vi "MainT4.vi"() -> ()   [LabVIEW 2019]
uses:
  <instrlib>/niDMM/nidmm.llb/niDMM Function.ctl
  <instrlib>/niDMM/nidmm.llb/niDMM Resolution in Digits.ctl
  <extravilib>/ChannelInstances/Tag-bool/Write With Abort.vi
  <extravilib>/ChannelInstances/Tag-bool/Read With Abort.vi
  <extravilib>/ChannelInstances/Tag-bool/Instantiate.vi
  <extravilib>/ChannelInstances/Tag-bool/EndpointRead.vi
  <extravilib>/ChannelInstances/Tag-bool/Endpoint.vi
  <extravilib>/ChannelInstances/Tag-bool.lvlib
panel:
  in  "stop program":bool
  in  "Tab Control":T1(tab)
  out "Waveform Chart 2":cluster{dbl, dbl, dbl}(graph)={9900000000.0, 100000.0, 100000.0}
  in  "Recieve Data":bool=TRUE
  in  "termination char\n(0xA = '\\n' = LF)":u8=13 format="%.0x"
  in  "VISA resource name":refnum<visa-resource-name>="COM3"
  out "time between obtaining data (ms)  (P)":u32
  out "output cluster":cluster{dbl, dbl, dbl}
  out "Waveform Chart 4":T2(graph)
  in  "physical channels":tag="PXI1Slot2/ai0:5"
  in  "resistance configuration":i32(ring)=4 items=["2-Wire"=2, "3-Wire"=3, "4-Wire"=4]
  out "time between obtaining data (ms) (T)":u32
  out "data":dbl[](array[numeric]) format="%0.2f"
  out "Waveform Chart 3":dbl(graph)
  in  "Instrument Descriptor":refnum<k15>="PXI1Slot4"
  in  "Function":T3
  in  "Resolution in Digits":T4=5.5 items=["3 1/2"=3.5, "4 1/2"=4.5, "5 1/2"=5.5, "6 1/2"=6.5, "7 1/2"=7.5]
  in  "Range (Volts)":dbl=10.0 format="%.2p"
  out "Over Range?":bool
  out "time between obtaining data (ms) (v/c)":u32
  out "Measurement (Volts)":dbl caption="Value" format="%_5p"
  in  "Self-Calibrate Multimeter at the beginning?":bool
  # "NEGRO bateria"
  # "BLANCO platina"
  # "VERDE fuente"
  # "AZUL MCU"
  # "AMARILLO AMBIENTE"
  # "ROJO BATERIA RELOJ"
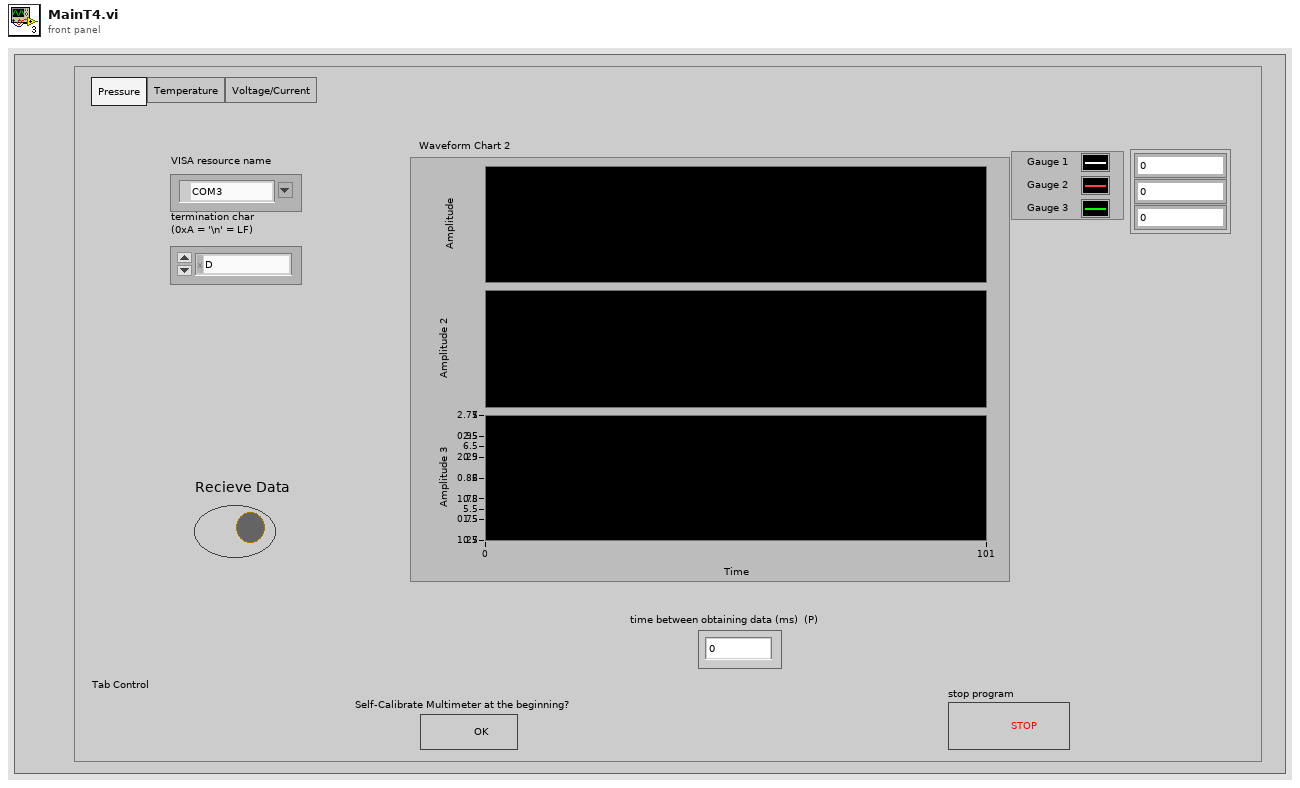
[diagram p1: front panel]
types:
  T1 = enum32{"Pressure", "Temperature", "Voltage/Current"}
  T2 = cluster{"data[0]":dbl, "data[1]":dbl, "data[2]":dbl, "data[3]":dbl, "data[4]":dbl, "data[5]":dbl, "data[6]":dbl, "data[7]":dbl, "data[8]":dbl}
  T3 = typedef "niDMM Function.ctl" = enum16{"DC Volts", "AC Volts", "DC Current", "AC Current", "2-wire Resistance", "4-wire Resistance", "Diode", "Frequency", "Period", "AC Volts DC Coupled", "Capacitance", "Inductance", "Temperature"}
  T4 = typedef "niDMM Resolution in Digits.ctl" = dbl
  T5 = typedef "Tag-bool.lvlib/))Channel.ctl" = refnum<queue>
  T6 = enum16{"open", "replace", "create", "open or create", "replace or create", "replace or create with confirmation"}
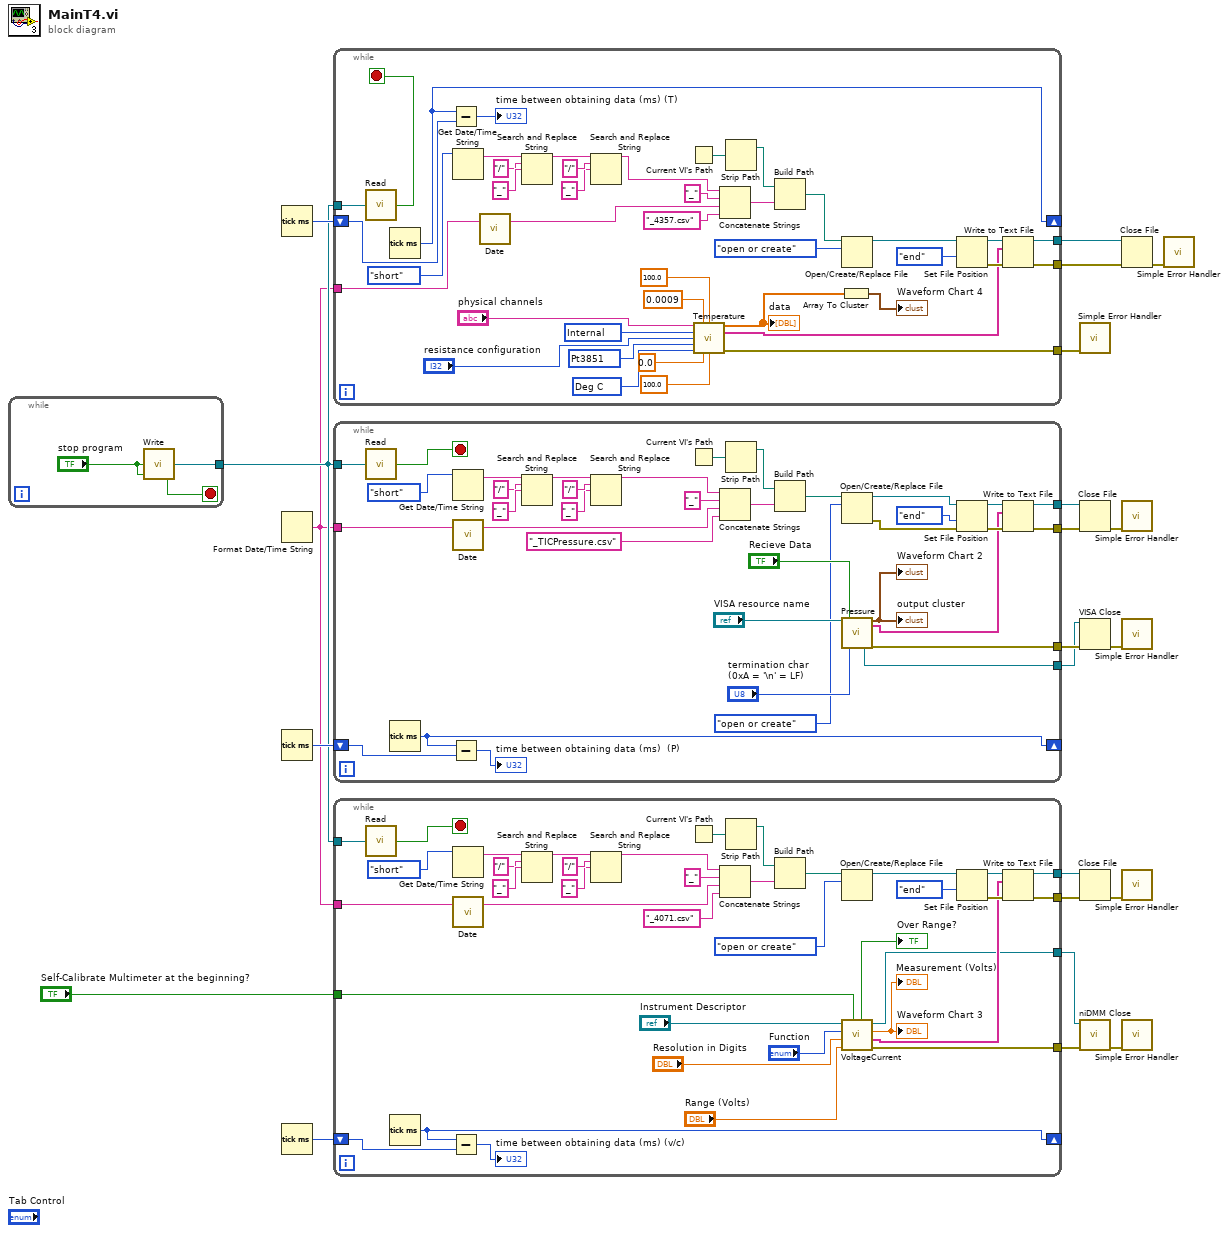
[diagram p0: block diagram]
diagram:
  n1 = while {
    tunnel: [w23] -> w3
    stop <- "stop program" stop-if-true
    n2 = call <extravilib>:"Write.vi"("element"="stop program") -> ("channel"=w23:T5)  [unwired: 1 out]
  }
  n3 = Tick Count (ms)() -> (millisecond timer value=w20:u32)
  n4 = Format Date/Time String() -> (date/time string=w1:string)  [unwired: 3 in]
  n5 = Tick Count (ms)() -> (millisecond timer value=w21:u32)
  n6 = Tick Count (ms)() -> (millisecond timer value=w22:u32)
  n7 = while {
    tunnel: [w48] -> w16
    tunnel: [w47] -> w4
    tunnel: [w46] -> w5
    shift-right: [w43] -> _
    shift-left: w20 -> [w44]
    tunnel: w3 -> [w40]
    tunnel: w1 -> [w28]
    stop <- w39 stop-if-true
    w51 = 10143 items=["Deg C"=10143, "Deg F"=10144, "Kelvins"=10325, "Deg R"=10145, "From Custom Scale"=10065] ("units")
    w52 = 10071 items=["Pt3750"=12481, "Pt3851"=10071, "Pt3911"=12482, "Pt3916"=10069, "Pt3920"=10053, "Pt3928"=12483, "Custom"=10137] ("rtd type")
    w53 = 10200 items=["Internal"=10200, "External"=10167, "None"=10230] ("current excitation source")
    n8 = call <extravilib>:"Read.vi"("channel"=w40) -> ("element"=w39:bool)  [unwired: 1 in, 1 out]
    n9 = Tick Count (ms)() -> (millisecond timer value=w43:u32)
    n10 = Subtract(x=w43, y=w44) -> (x-y=→"time between obtaining data (ms) (T)":u32)
    n11 = Get Date/Time String(date format (0)=enum16{"short", "long", "abbreviated"}."short") -> (date string=w34:string)  [unwired: 2 in, 1 out]
    n12 = call "Date.vi"("Format Date/Time String"=w28) -> ("result string"=w25:string)  [unwired: 2 in]
    n13 = Search and Replace String(input string=w34, search string="/", replace string="_" ("replace string (\"\")")) -> (result string=w37:string)  [unwired: 5 in, 3 out]
    n14 = Search and Replace String(input string=w37, search string="/", replace string="_" ("replace string (\"\")")) -> (result string=w31:string)  [unwired: 5 in, 3 out]
    n15 = Current VI's Path() -> (path=w59:path)
    n16 = call "Temperature.vi"("physical channels"="physical channels", "current excitation value"=0.0009, "r0"=100.0, "current excitation source"=w53, "resistance configuration"="resistance configuration", "rtd type"=w52, "units"=w51, "minimum value"=0.0, "maximum value"=100.0) -> ("data"=w42:dbl[], "output array"=w29:string[], "error out"=w48:errorcluster)  [unwired: 4 in]
    "data" <- w42
    n17 = Concatenate Strings(w31, "_" ("string"), w25, "_4357.csv" ("string")) -> (w30:string)
    n18 = Strip Path(path=w59) -> (stripped path=w58:path)  [unwired: 1 out]
    n19 = Build Path(base path=w58, name or relative path=w30) -> (appended path=w65:path)
    n20 = Array To Cluster(array=w42) -> (cluster=→"Waveform Chart 4":T2)
    n21 = Open/Create/Replace File(file path (use dialog)=w65, operation (0:open)=T6."open or create") -> (refnum out=w62:refnum<file>)  [unwired: 4 in, 2 out]
    n22 = Set File Position(refnum=w62, from (0:start)=enum16{"start", "end", "current"}."end") -> (refnum out=w63:refnum<file>, error out=w64:errorcluster)  [unwired: 2 in]
    n23 = Write to Text File(file (use dialog)=w63, text=w29, error in=w64) -> (refnum out=w47:refnum<file>, error out=w46:errorcluster)  [unwired: 1 in, 1 out]
  }
  n24 = while {
    tunnel: [w87] -> w7
    tunnel: [w86] -> w8
    tunnel: [w85] -> w9
    tunnel: [w84] -> w10
    shift-right: [w81] -> _
    shift-left: w21 -> [w82]
    tunnel: w3 -> [w80]
    tunnel: w1 -> [w69]
    stop <- w79 stop-if-true
    n25 = call <extravilib>:"Read.vi"("channel"=w80) -> ("element"=w79:bool)  [unwired: 1 in, 1 out]
    n26 = Tick Count (ms)() -> (millisecond timer value=w81:u32)
    n27 = Subtract(x=w81, y=w82) -> (x-y=→"time between obtaining data (ms)  (P)":u32)
    n28 = Get Date/Time String(date format (0)=enum16{"short", "long", "abbreviated"}."short") -> (date string=w74:string)  [unwired: 2 in, 1 out]
    n29 = call "Date.vi"("Format Date/Time String"=w69) -> ("result string"=w67:string)  [unwired: 2 in]
    n30 = Search and Replace String(input string=w74, search string="/", replace string="_" ("replace string (\"\")")) -> (result string=w77:string)  [unwired: 5 in, 3 out]
    n31 = Search and Replace String(input string=w77, search string="/", replace string="_" ("replace string (\"\")")) -> (result string=w71:string)  [unwired: 5 in, 3 out]
    n32 = Current VI's Path() -> (path=w90:path)
    n33 = Concatenate Strings(w71, "_" ("string"), w67, "_TICPressure.csv" ("string")) -> (w70:string)
    n34 = Strip Path(path=w90) -> (stripped path=w89:path)  [unwired: 1 out]
    n35 = Build Path(base path=w89, name or relative path=w70) -> (appended path=w97:path)
    n36 = Open/Create/Replace File(file path (use dialog)=w97, operation (0:open)=T6."open or create") -> (refnum out=w94:refnum<file>, error out=w91:errorcluster)  [unwired: 4 in, 1 out]
    n37 = call "Pressure.vi"("VISA resource name"="VISA resource name", "Recieve Data"="Recieve Data", "termination char\n(0xA = '\\n' = LF)"="termination char\n(0xA = '\\n' = LF)") -> ("VISA resource name out"=w87:refnum<visa-resource-name>, "output cluster"=→"Waveform Chart 2" →"output cluster":cluster{dbl, dbl, dbl}, "output array"=w88:string[], "error out"=w86:errorcluster)  [unwired: 10 in, 3 out]
    n38 = Set File Position(refnum=w94, from (0:start)=enum16{"start", "end", "current"}."end", error in=w91) -> (refnum out=w95:refnum<file>, error out=w96:errorcluster)  [unwired: 1 in]
    n39 = Write to Text File(file (use dialog)=w95, text=w88, error in=w96) -> (refnum out=w85:refnum<file>, error out=w84:errorcluster)  [unwired: 1 in, 1 out]
  }
  n40 = while {
    tunnel: "Self-Calibrate Multimeter at the beginning?" -> [w135]
    tunnel: [w123] -> w11
    tunnel: [w122] -> w12
    tunnel: [w121] -> w14
    tunnel: [w120] -> w15
    shift-right: [w117] -> _
    shift-left: w22 -> [w118]
    tunnel: w3 -> [w116]
    tunnel: w1 -> [w105]
    stop <- w115 stop-if-true
    n41 = call <extravilib>:"Read.vi"("channel"=w116) -> ("element"=w115:bool)  [unwired: 1 in, 1 out]
    n42 = Tick Count (ms)() -> (millisecond timer value=w117:u32)
    n43 = Subtract(x=w117, y=w118) -> (x-y=→"time between obtaining data (ms) (v/c)":u32)
    n44 = Get Date/Time String(date format (0)=enum16{"short", "long", "abbreviated"}."short") -> (date string=w110:string)  [unwired: 2 in, 1 out]
    n45 = call "Date.vi"("Format Date/Time String"=w105) -> ("result string"=w103:string)  [unwired: 2 in]
    n46 = Search and Replace String(input string=w110, search string="/", replace string="_" ("replace string (\"\")")) -> (result string=w113:string)  [unwired: 5 in, 3 out]
    n47 = Search and Replace String(input string=w113, search string="/", replace string="_" ("replace string (\"\")")) -> (result string=w107:string)  [unwired: 5 in, 3 out]
    n48 = Current VI's Path() -> (path=w126:path)
    n49 = Concatenate Strings(w107, "_" ("string"), w103, "_4071.csv" ("string")) -> (w106:string)
    n50 = Strip Path(path=w126) -> (stripped path=w125:path)  [unwired: 1 out]
    n51 = Build Path(base path=w125, name or relative path=w106) -> (appended path=w132:path)
    n52 = Open/Create/Replace File(file path (use dialog)=w132, operation (0:open)=T6."open or create") -> (refnum out=w129:refnum<file>)  [unwired: 4 in, 2 out]
    n53 = call "VoltageCurrent.vi"("Self-Calibrate at the beginning?"=w135, "Range (Volts)"="Range (Volts)", "Resolution in Digits"="Resolution in Digits", "Function"="Function", "Instrument Descriptor"="Instrument Descriptor") -> ("error out"=w120:errorcluster, "output array"=w124:string[], "Measurement (Volts)"=→"Waveform Chart 3" →"Measurement (Volts)":dbl, "instrument handle out"=w121:refnum<k15>, "Over Range?"=→"Over Range?":bool)  [unwired: 2 in]
    n54 = Set File Position(refnum=w129, from (0:start)=enum16{"start", "end", "current"}."end") -> (refnum out=w130:refnum<file>, error out=w131:errorcluster)  [unwired: 2 in]
    n55 = Write to Text File(file (use dialog)=w130, text=w124, error in=w131) -> (refnum out=w123:refnum<file>, error out=w122:errorcluster)  [unwired: 1 in, 1 out]
  }
  n56 = call <vilib>:"Simple Error Handler.vi"("error in (no error)"=w16) -> ()  [unwired: 1 in, 8 out]
  n57 = Close File(refnum=w9, error in=w10) -> (error out=w18:errorcluster)  [unwired: 1 out]
  n58 = VISA Close(VISA resource name=w7, error in (no error)=w8) -> (error out=w17:errorcluster)
  n59 = Close File(refnum=w11, error in=w12) -> (error out=w19:errorcluster)  [unwired: 1 out]
  n60 = call <instrlib>:"niDMM Close.vi"("error in (no error)"=w15, "instrument handle"=w14) -> ("error out"=w13:errorcluster)  [unwired: 9 in]
  n61 = Close File(refnum=w4, error in=w5) -> (error out=w6:errorcluster)  [unwired: 1 out]
  n62 = call <vilib>:"Simple Error Handler.vi"("error in (no error)"=w18) -> ()  [unwired: 1 in, 8 out]
  n63 = call <vilib>:"Simple Error Handler.vi"("error in (no error)"=w17) -> ()  [unwired: 4 in, 5 out]
  n64 = call <vilib>:"Simple Error Handler.vi"("error in (no error)"=w19) -> ()  [unwired: 2 in, 7 out]
  n65 = call <vilib>:"Simple Error Handler.vi"("error in (no error)"=w13) -> ()  [unwired: 4 in, 5 out]
  n66 = call <vilib>:"Simple Error Handler.vi"("error in (no error)"=w6) -> ()  [unwired: 1 in, 8 out]
